vi "File or Folder Exist.vi"(5 "file or folder":path) -> (2 "exist?":bool)   [LabVIEW 2020]
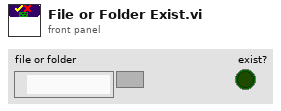
[diagram p1: front panel]
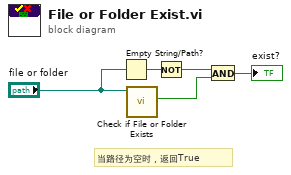
[diagram p0: block diagram]
diagram:
  # "当路径为空时，返回True"
  n1 = Empty String/Path?(string/path="file or folder") -> (empty?=w4:bool)
  n2 = call <vilib>:"Check if File or Folder Exists.vi"("path"="file or folder") -> ("file or folder exists?"=w2:bool)  [unwired: 8 in, 2 out]
  n3 = Not(x=w4) -> (.not. x?=w3:bool)
  n4 = And(x=w3, y=w2) -> (x .and. y?=→"exist?":bool)
